vi "S2C_Access_ReadAppCfg.vi"(8 "Error In":errorcluster) -> (0 "Error Out":errorcluster)   [LabVIEW 2015]
doc: "Reads the data contained within the Settings file and loads the data into VI specific global variables."
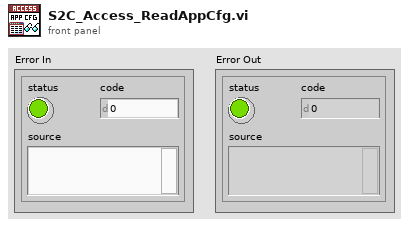
[diagram p1: front panel]
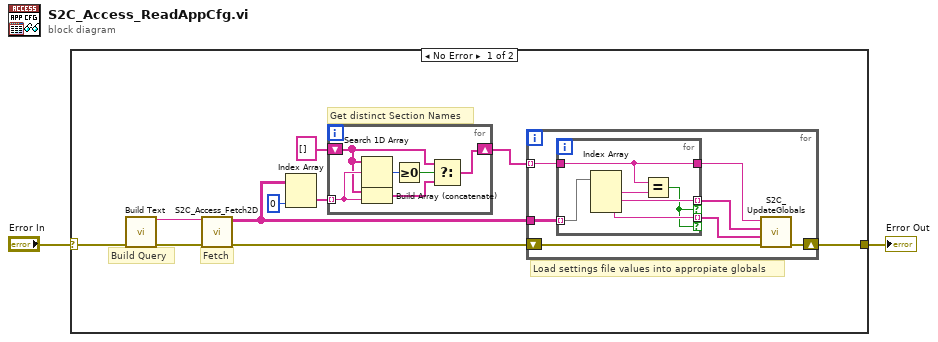
[diagram p0: block diagram]
diagram:
  n1 = case shown="No Error" "Error In" {
    selector: "Error In" -> [w3 w32]
    tunnel: [w4 w32] -> w1
    frame No Error {
      # "Load settings file values into appropiate globals"
      # "Get distinct Section Names"
      # "Fetch"
      # "Build Query"
      n2 = call "Build Text"("error in (no error)"=w3) -> ("Result"=w10:string, "error out"=w12:errorcluster)  [unwired: 13 in]
      n3 = call "S2C_Access_Fetch2D.vi"("Error In"=w12, "Query"=w10) -> ("Error Out"=w11:errorcluster, "Data"=w9:string[][])  [unwired: 8 in]
      n4 = Index Array(array=w9, index (col)=0 ("disabled index (col)")) -> (element=w7:string[])  [unwired: 1 in]
      n5 = for {
        shift-right: [w13] -> w5
        shift-left: string[] [] -> [w15]
        tunnel: w7 -> [w16] mode=indexing
        n6 = Search 1D Array(1D array=w15, element=w16) -> (index of element=w18:i32)  [unwired: 1 in]
        n7 = Build Array (concatenate)(w15, w16) -> (w14:string[])
        n8 = Greater Or Equal To 0?(x=w18) -> (x >= 0?=w17:bool)
        n9 = Select(t=w15, s=w17, f=w14) -> (s? t:f=w13:string[])
      }
      n10 = for {
        tunnel: w9 -> [w25]
        shift-right: [w23] -> w4
        shift-left: w11 -> [w24]
        tunnel: w5 -> [w20] mode=indexing
        n11 = for {
          tunnel: w25 -> [w31] mode=indexing
          tunnel: [w29] -> w22 mode=indexing if=w27
          tunnel: [w28] -> w21 mode=indexing if=w27
          tunnel: w20 -> [w26]
          tunnel: [w26] -> w19
          n12 = Index Array(array=w31) -> (element #1=w30:string, element #2=w29:string, element #3=w28:string)  [unwired: 3 in]
          n13 = Equal?(x=w26, y=w30) -> (x = y?=w27:bool)
        }
        n14 = call "S2C_UpdateGlobals.vi"("Error In"=w24, "Values"=w21, "Keys"=w22, "Section"=w19) -> ("Error Out"=w23:errorcluster)  [unwired: 7 in]
      }
    }
    frame Error {
    }
  }
  "Error Out" <- w1
